vi "TOP-配置文件模块.vi"(8 "error in (no error)":errorcluster caption="错误输入（无错误）", 11 "输入":T4) -> (0 "error out":errorcluster caption="错误输出", 3 "配置文件":T1 {"定时配置-自动导出"."定时配置-自动导出"."间隔" min=1; "定时配置-累积分段"."间隔" min=1})   [LabVIEW 2017]
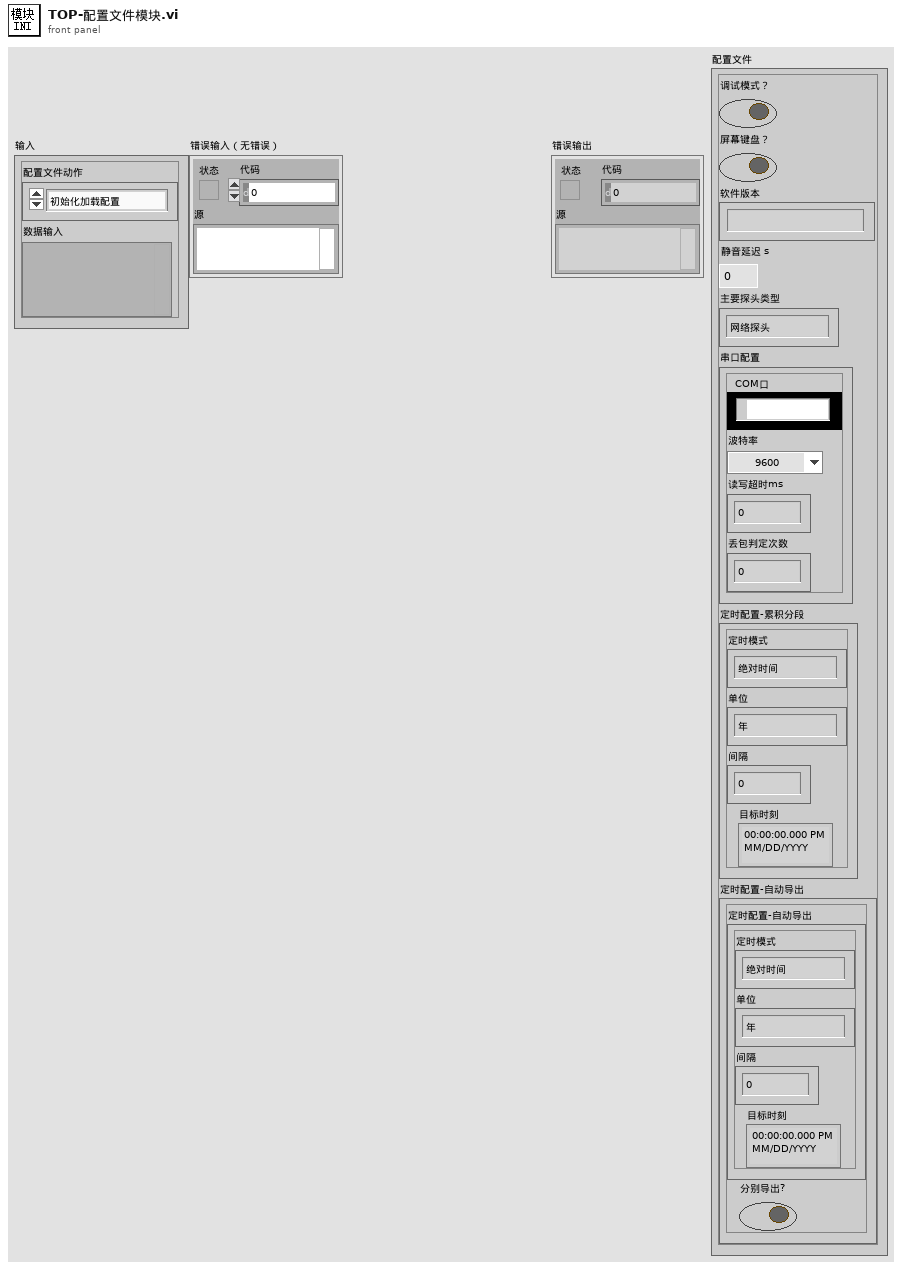
[diagram p1: front panel]
types:
  T1 = typedef "簇-配置文件内容.ctl" = cluster{"调试模式？":bool, "屏幕键盘？":bool, "软件版本":string, "静音延迟 s":u16, "主要探头类型":T2, "串口配置":cluster{"COM口":refnum<visa-resource-name>, "波特率":enum16{"9600", "19200"}, "读写超时ms":i16, "丢包判定次数":i16}, "定时配置-累积分段":T3, "定时配置-自动导出":cluster{"定时配置-自动导出":T3, "分别导出?":bool}}
  T2 = typedef "枚举-主要探头类型.ctl" = enum16{"网络探头", "串口探头"}
  T3 = typedef "簇-定时配置.ctl" = cluster{"定时模式":enum16{"绝对时间", "相对时间"}, "单位":enum16{"年", "月", "日", "时", "分"}, "间隔":u8, "目标时刻":timestamp}
  T4 = typedef "簇-输入.ctl" = cluster{"配置文件动作":T5, "数据输入":variant}
  T5 = typedef "枚举-配置文件动作.ctl" = enum16{"初始化加载配置", "读取配置", "写入-屏幕键盘", "写入-静音延迟", "写入-主要探头类型", "写入-串口配置", "写入-累积定时", "写入-导出定时", "保存配置到文件"}
  T6 = cluster{"COM口":refnum<visa-resource-name>, "波特率":enum16{"9600", "19200"}, "读写超时ms":i16, "丢包判定次数":i16}
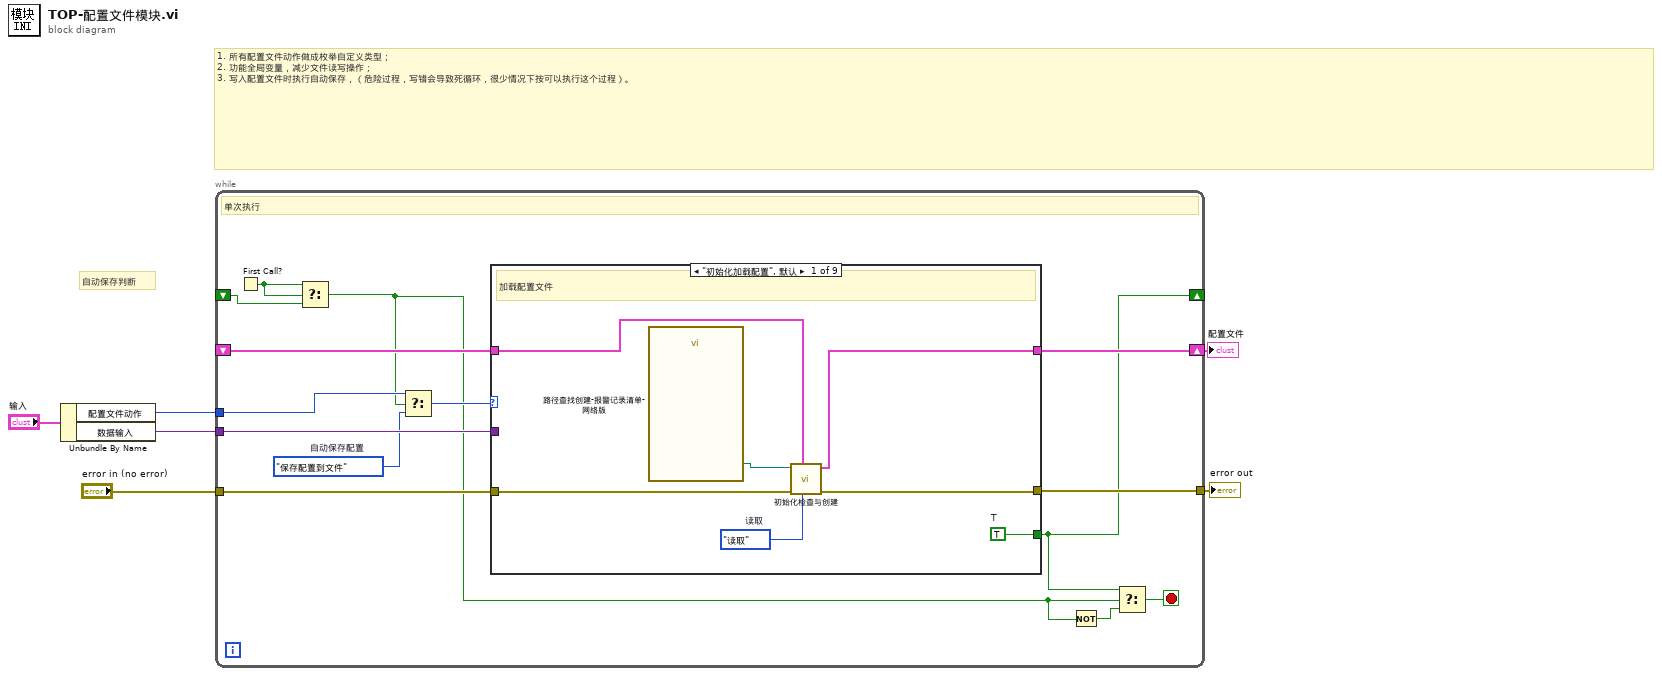
[diagram p0: block diagram]
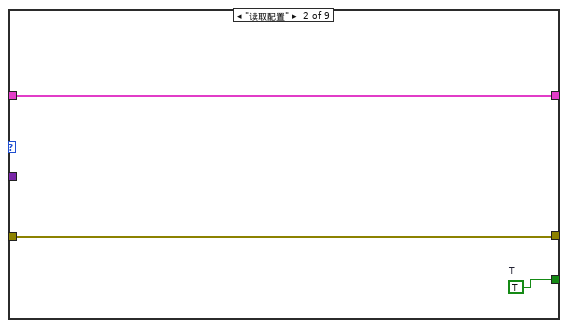
[diagram p2: hidden frame]
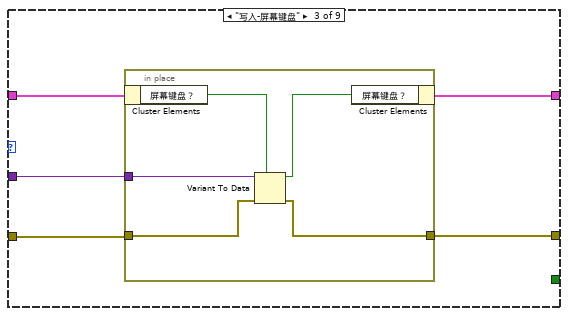
[diagram p3: hidden frame]
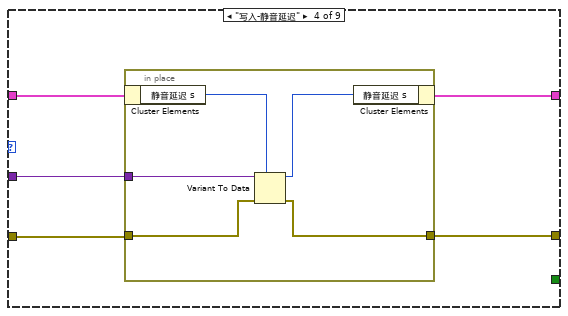
[diagram p4: hidden frame]
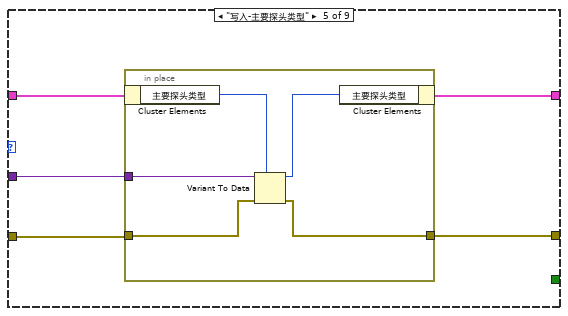
[diagram p5: hidden frame]
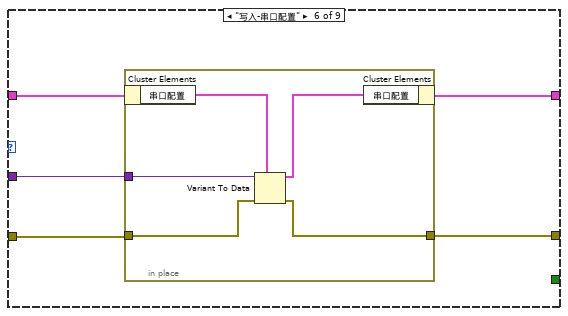
[diagram p6: hidden frame]
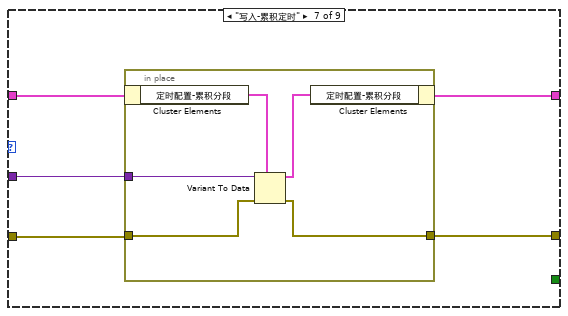
[diagram p7: hidden frame]
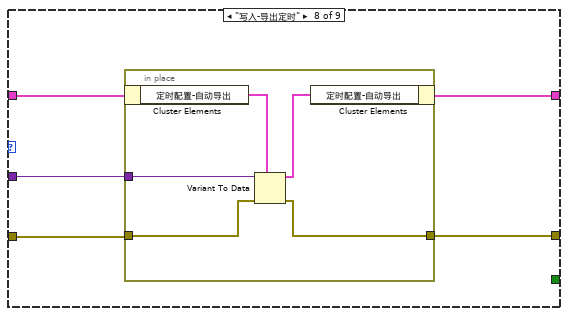
[diagram p8: hidden frame]
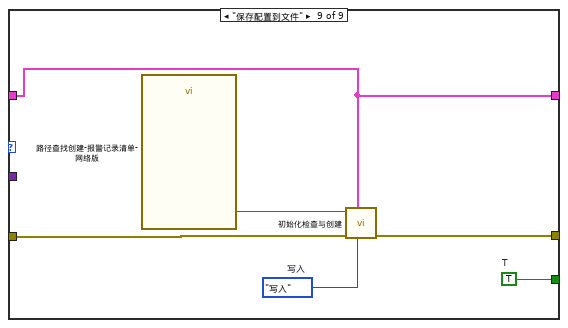
[diagram p9: hidden frame]
diagram:
  # "1. 所有配置文件动作做成枚举自定义类型；\n2. 功能全局变量，减少文件读写操作；\n3. 写入配置文件时执行自动保存，（危险过程，写错会导致死循环，很少情况下按可以执行这个过程）。"
  # "自动保存判断"
  n1 = Unbundle By Name("输入") -> ("配置文件动作"=w5:T5, "数据输入"=w2:variant)
  n2 = while {
    tunnel: w5 -> [w15]
    shift-right: [w19] -> w1
    shift-left: _ -> [w20]
    tunnel: "error in (no error)" -> [w18]
    tunnel: [w17] -> w3
    tunnel: w2 -> [w16]
    shift-right: [w11] -> _
    shift-left: _ -> [w12]
    stop <- w10 stop-if-true
    w14 = 枚举-配置文件动作."保存配置到文件"  # 自动保存配置
    # "单次执行"
    n3 = First Call?() -> (First Call?: T/F=w9:bool)
    n4 = Select(t=w9, s=w9, f=w12) -> (s? t:f=w8:bool)
    n5 = Select(t=w15, s=w8, f=w14) -> (s? t:f=w13:T5)
    n6 = case shown="\"初始化加载配置\", 默认" w13 {
      tunnel: w20 -> [w23 w30 w32 w42 w52 w62 w72 w82 w92]
      tunnel: [w26 w30 w31 w41 w51 w61 w71 w81 w92] -> w19
      tunnel: w18 -> [w25 w29 w34 w44 w54 w64 w74 w84 w95]
      tunnel: [w24 w29 w33 w43 w53 w63 w73 w83 w94] -> w17
      tunnel: w16 -> [_ _ w35 w45 w55 w65 w75 w85 _]
      tunnel: [w21 w28 _ _ _ _ _ _ w91] -> w11
      frame "初始化加载配置", Default {
        w21 = TRUE  # T
        w22 = enum16{"读取", "写入"}."读取"  # 读取
        # "加载配置文件"
        n7 = call "路径查找创建-报警记录清单-网络版.vi"() -> ("配置文件"=w27:path)  [unwired: 2 in, 13 out]
        n8 = call "初始化检查与创建.vi"("模式(读取)"=w22, "配置文件 i"=w23, "error in (no error)"=w25, "配置文件路径"=w27) -> ("error out"=w24:errorcluster, "配置文件 o"=w26:T1)  [unwired: 6 in]
      }
      frame "读取配置" {
        w28 = TRUE  # T
      }
      frame "写入-屏幕键盘" {
        n9 = in-place {
          in-place-border: w35 -> [w40]
          in-place-border: w34 -> [w39]
          in-place-border: [w38] -> w33
          n10 = in-place-cluster #1(w32) -> ("屏幕键盘？"=w37:bool)
          n11 = Variant To Data(error in=w39, type=w37, Variant=w40) -> (data=w36:bool, error out=w38:errorcluster)
          n12 = in-place-cluster #1("屏幕键盘？"=w36) -> (w31:T1)
        }
      }
      frame "写入-静音延迟" {
        n13 = in-place {
          in-place-border: w45 -> [w50]
          in-place-border: w44 -> [w49]
          in-place-border: [w48] -> w43
          n14 = in-place-cluster #2(w42) -> ("静音延迟 s"=w47:u16)
          n15 = Variant To Data(error in=w49, type=w47, Variant=w50) -> (data=w46:u16, error out=w48:errorcluster)
          n16 = in-place-cluster #2("静音延迟 s"=w46) -> (w41:T1)
        }
      }
      frame "写入-主要探头类型" {
        n17 = in-place {
          in-place-border: w55 -> [w60]
          in-place-border: w54 -> [w59]
          in-place-border: [w58] -> w53
          n18 = in-place-cluster #3(w52) -> ("主要探头类型"=w57:T2)
          n19 = Variant To Data(error in=w59, type=w57, Variant=w60) -> (data=w56:T2, error out=w58:errorcluster)
          n20 = in-place-cluster #3("主要探头类型"=w56) -> (w51:T1)
        }
      }
      frame "写入-串口配置" {
        n21 = in-place {
          in-place-border: w65 -> [w70]
          in-place-border: w64 -> [w69]
          in-place-border: [w68] -> w63
          n22 = in-place-cluster #4(w62) -> ("串口配置"=w67:T6)
          n23 = Variant To Data(error in=w69, type=w67, Variant=w70) -> (data=w66:T6, error out=w68:errorcluster)
          n24 = in-place-cluster #4("串口配置"=w66) -> (w61:T1)
        }
      }
      frame "写入-累积定时" {
        n25 = in-place {
          in-place-border: w75 -> [w80]
          in-place-border: w74 -> [w79]
          in-place-border: [w78] -> w73
          n26 = in-place-cluster #5(w72) -> ("定时配置-累积分段"=w77:T3)
          n27 = Variant To Data(error in=w79, type=w77, Variant=w80) -> (data=w76:T3, error out=w78:errorcluster)
          n28 = in-place-cluster #5("定时配置-累积分段"=w76) -> (w71:T1)
        }
      }
      frame "写入-导出定时" {
        n29 = in-place {
          in-place-border: w85 -> [w90]
          in-place-border: w84 -> [w89]
          in-place-border: [w88] -> w83
          n30 = in-place-cluster #6(w82) -> ("定时配置-自动导出"=w87:cluster{"定时配置-自动导出":T3, "分别导出?":bool})
          n31 = Variant To Data(error in=w89, type=w87, Variant=w90) -> (data=w86:cluster{"定时配置-自动导出":T3, "分别导出?":bool}, error out=w88:errorcluster)
          n32 = in-place-cluster #6("定时配置-自动导出"=w86) -> (w81:T1)
        }
      }
      frame "保存配置到文件" {
        w91 = TRUE  # T
        w93 = enum16{"读取", "写入"}."写入"  # 写入
        n33 = call "路径查找创建-报警记录清单-网络版.vi"() -> ("配置文件"=w96:path)  [unwired: 2 in, 13 out]
        n34 = call "初始化检查与创建.vi"("模式(读取)"=w93, "配置文件 i"=w92, "error in (no error)"=w95, "配置文件路径"=w96) -> ("error out"=w94:errorcluster)  [unwired: 6 in, 1 out]
      }
    }
    n35 = Not(x=w8) -> (.not. x?=w7:bool)
    n36 = Select(t=w11, s=w8, f=w7) -> (s? t:f=w10:bool)
  }
  "error out" <- w3
  "配置文件" <- w1
